vi "ColorToNeoPixel.vi"(10 "Color Box":u32(colorbox), 11 "Lightness":u8) -> (1 "NeoPBlue":u8=250 format="%.0x", 2 "NeoPGreen":u8=250 format="%.0x", 3 "NeoPRed":u8=250 format="%.0x")   [LabVIEW 2020, in "CTI-Peripheral.lvlib" / "AdaFruit-Seesaw.lvclass"]
uses:
  AdaFruit-Seesaw.lvclass
panel:
  out "blue":u8=250 format="%.0x"
  out "Green":u8=250 format="%.0x"
  out "Red":u8=250 format="%.0x"
  # "Input"
  # "Local"
  # "Output"
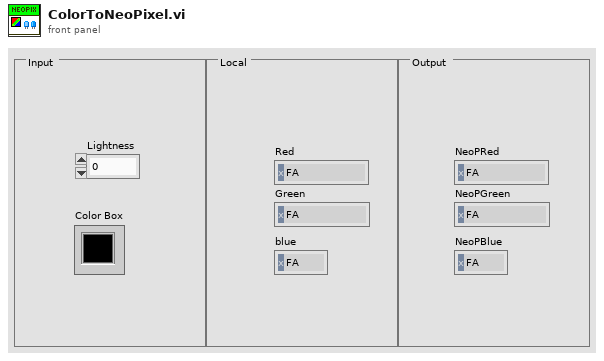
[diagram p1: front panel]
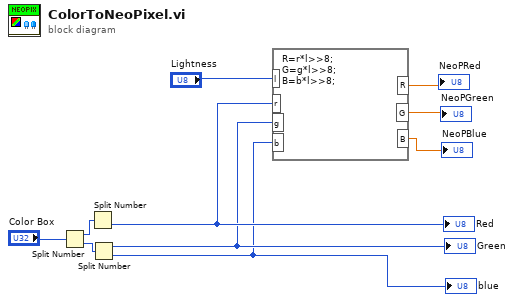
[diagram p0: block diagram]
diagram:
  n1 = Split Number(x="Color Box") -> (hi(x)=w9:u16, lo(x)=w10:u16)
  n2 = Split Number(x=w9) -> (lo(x)=w5:u8)  [unwired: 1 out]
  "Red" <- w5
  n3 = Split Number(x=w10) -> (hi(x)=w4:u8, lo(x)=w3:u8)
  "Green" <- w4
  "blue" <- w3
  n4 = formula code="R=r*l>>8;\nG=g*l>>8;\nB=b*l>>8;"("l"="Lightness", "r"=w5, "g"=w4, "b"=w3) -> ("R"=→"NeoPRed":dbl, "G"=→"NeoPGreen":dbl, "B"=→"NeoPBlue":dbl)
